vi "Teleop.vi"(10 "Match Info":T3={"Autonomous Elapsed Seconds"=0.0, "TeleOp Elapsed Seconds"=0.0, "Disabled Elapsed Seconds"=0.0, "Visited Autonomous"=FALSE, "Visited TeleOp"=FALSE, "Visited Disabled"=FALSE, "Autonomous Settings"={"Autonomous Style"=enum."Independent", "VI Refnum"=refnum}}, 11 "Call Context":T4) -> ()   [LabVIEW 2012]
doc: "This VI is called for each TeleOp packet received from the DS where the robot is not disabled. It is often used to read from the joysticks and update I/O or to update setpoints for timed control loops. It should complete and return within 20 milliseconds or it may miss DS packets."
uses:
  <vilib>/Rock Robotics/WPI/DriverStation/WPI_DriverStationDerivedRobotMode.ctl
  <vilib>/Rock Robotics/WPI/DriverStation/WPI_DriverStationMatch Info.ctl
  Control 1.ctl
  Robot Global Data.vi
  <vilib>/addons/control/pid/pid.llb/PID Output Rate Limiter (DBL).vi
  <vilib>/Rock Robotics/WPI/Joystick/WPI_JoystickGetSetRefNum.vi
  <vilib>/ptbypt/NI_PtbyPt.lvlib
  <vilib>/addons/control/pid/NI_PID_pid.lvlib
panel:
  in  "rate":dbl=500.0 format="%.2f"
  in  "ShooterTolerance":dbl=35.0
  out "RPM":dbl
  out "Pitch":dbl
  out "Enum":enum16{"Move Motor", "Engaged", "Disengaged"}(ring)
  in  "Break Disengaged":i32
  in  "Retract SH":dbl=-0.1
  in  "Time to retract motor":dbl=0.2
  in  "Break Engaged":i32=120
  in  "Test Pitch":bool
  in  "Test RPM":bool
  out "Load":bool
  in  "Reset Climb Encoder":bool
  out "Personality":string
  out "Climb Amps":dbl(graph)
  in  "sample length":i32=50
  in  "Slow Mode Divider":dbl(knob)=1.6756203903545743 scale=0.0..2.0
  in  "Elev Loop Active":bool=TRUE
  in  "Elev Bump Quanta":dbl=0.5
  out "Elev Bump":dbl
  in  "Reset Elev Bumps":bool
  out "Elevator":T1(graph)
  out "ElevatorResponse":dbl
  in  "Elevator Control (deg)":dbl(knob)=30.506718325532383 scale=15.0..40.0 scale format="%#_3g"
  in  "Reset RPM Bumps":bool
  out "RPM Bump":i64
  in  "RPM Bump Quanta":dbl=100.0
  in  "Reset Gyro":bool
  out "Climb Current":dbl
  out "Gyro Angle":dbl
  out "Elevator Encoder Volts":dbl
  out "Compressor Switch":bool
  out "Climb Encoder":dbl
  out "BB Prime":bool
  out "BB On Deck":bool
  out "Sky Hook Home":bool
  out "Drive Encoders":T1(graph)
  out "Drive Data":cluster{"Left":dbl, "Right":dbl}
  in  "Square":bool=TRUE
  in  "Which?":bool
  in  "Cheesy High & Low":T2=0.6 scale=0.0..1.0
  in  "Cheesy High":dbl(knob)=0.6 scale=0.0..1.0
  in  "Cheesy Low":dbl(knob)=0.6 scale=0.0..1.0
  in  "Quick Turn":T2=1.0 scale=0.0..1.0
  in  "Reset Encoder":bool
  out "Average Wheel Encoder":dbl
  out "Right Wheel Encoder":dbl
  out "Left Wheel Encoder":dbl
  out "Shooter RPM":cluster{dbl, "ShooterRpmResponse":dbl}(graph)
  out "Shooter RPM":dbl
  in  "Shooter RPM control":dbl(knob)=4201.533768386046 scale=0.0..5000.0
  out "Numeric 1":dbl(slide) scale=0.0..100.0
  out "Boolean 2":bool
  out "Boolean 1":bool
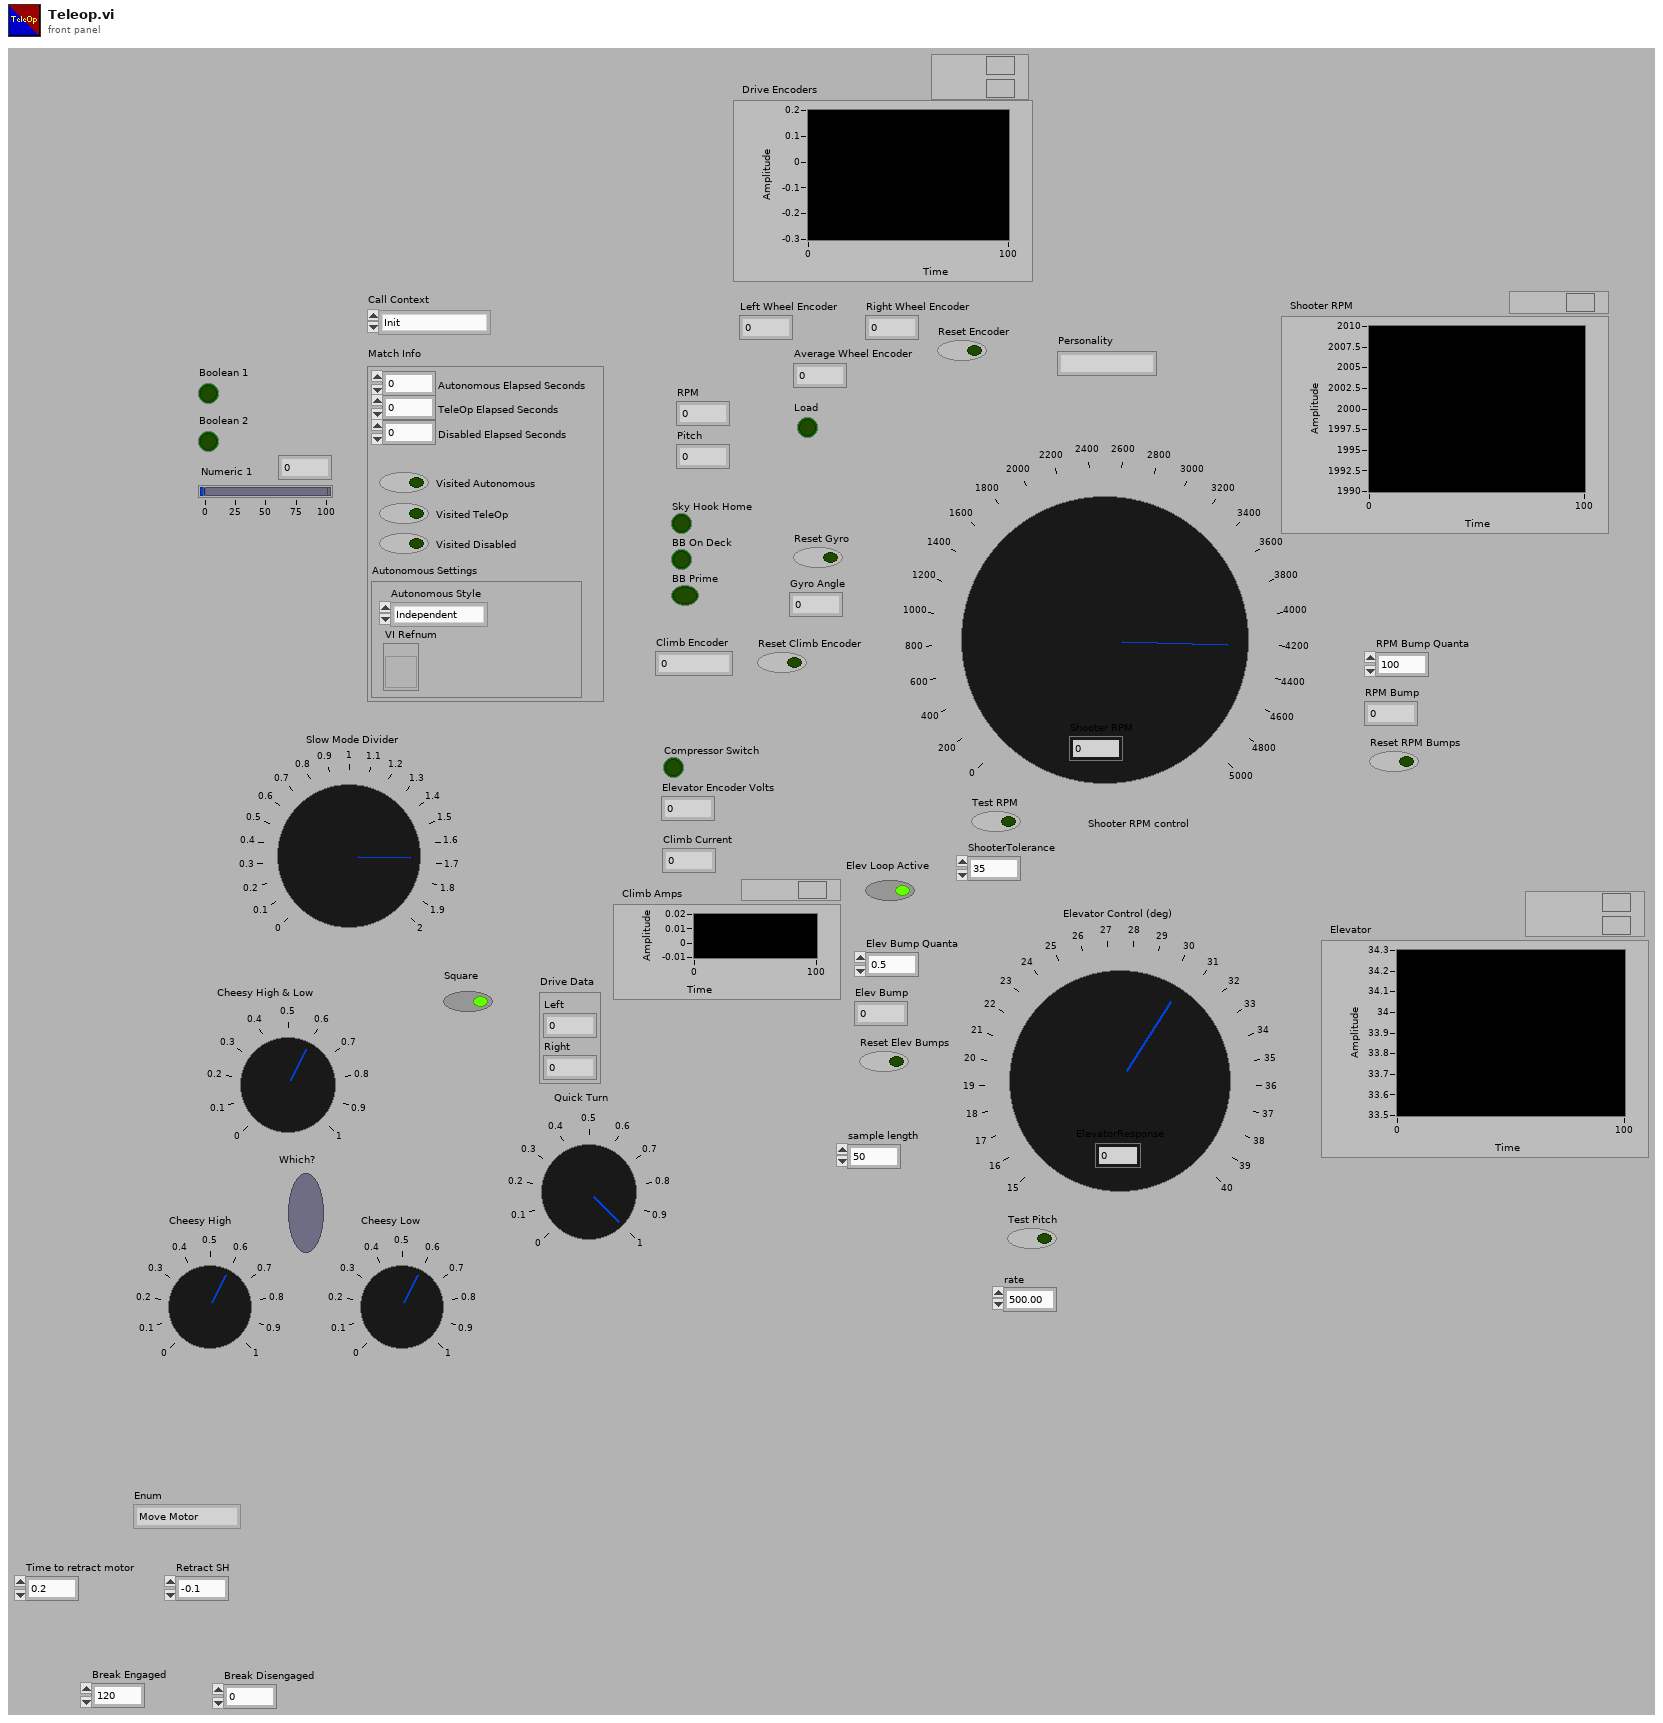
[diagram p1: front panel]
types:
  T1 = cluster{"Shooter RPM control":dbl, "ShooterRpmResponse":dbl}
  T2 = typedef "Control 1.ctl" = dbl
  T3 = typedef "WPI_DriverStationMatch Info.ctl" = cluster{"Autonomous Elapsed Seconds":dbl, "TeleOp Elapsed Seconds":dbl, "Disabled Elapsed Seconds":dbl, "Visited Autonomous":bool, "Visited TeleOp":bool, "Visited Disabled":bool, "Autonomous Settings":cluster{"Autonomous Style":enum16{"Iterative", "Independent"}, "VI Refnum":refnum<vi>}}
  T4 = typedef "WPI_DriverStationDerivedRobotMode.ctl" = enum16{"Init", "Execute", "Stop"}
  T5 = typedef "WPI_ServoDeviceRef.ctl" = cluster{"DeviceStatus":errorcluster, "Digital Module":T6, "PWM Channel":T7, "DeadBand":T8}
  T6 = typedef "FPGA_TypedefDigitalModule.ctl" = enum16{"Digital Module 1", "Digital Module 2"}
  T7 = typedef "FPGA_DIOPWMChannel.ctl" = enum8{"PWM 1", "PWM 2", "PWM 3", "PWM 4", "PWM 5", "PWM 6", "PWM 7", "PWM 8", "PWM 9", "PWM 10", "Invalid"}
  T8 = typedef "WPI_PWMDeadband.ctl" = cluster{"Name":string, "maxPositivePwm":i32, "minPositivePwm":i32, "centerPwm":i32, "maxNegativePwm":i32, "minNegativePwm":i32, "angularRange":u16}
  T9 = typedef "WPI_MotorControlDeviceRef.ctl" = cluster{"DeviceStatus":errorcluster, "Type":enum16{"PWM", "CAN"}, "PWM":cluster{"Digital Module":T6, "PWM Channel":T7, "DeadBand":T8}, "CAN":cluster{"Device Number":u8, "Control Mode":T10, "Semaphore":T11, "Max Vout":dbl}, "Invert":bool, "TransformRef":T12, "InvTransformRef":T12}
  T10 = typedef "WPI_CANJaguar_ControlMode.ctl" = enum8{"Percent VBus", "Current", "Speed", "Position", "Voltage"}
  T11 = typedef "Semaphore RefNum" = refnum<k1>
  T12 = typedef "WPI_PWMTransform_ConPane.ctl" = refnum<vi>
  T13 = typedef "WPI_JoystickDevRef.ctl" = cluster{"Device":T14}
  T14 = typedef "WPI_JoystickDeviceEnum.ctl" = enum16{"USB 1", "USB 2", "USB 3", "USB 4", "Kinect 1", "Kinect 2"}
  T15 = typedef "WPI_JoystickButtonState.ctl" = cluster{"Button 1":bool, "Button 2":bool, "Button 3":bool, "Button 4":bool, "Button 5":bool, "Button 6":bool, "Button 7":bool, "Button 8":bool, "Button 9":bool, "Button 10":bool, "Button 11":bool, "Button 12":bool}
  T16 = cluster{"axis 1 (x)":dbl, "axis 2 (y)":dbl, "axis 3 (throttle)":dbl, "axis 4":dbl, "axis 5":dbl, "axis 6":dbl}
  T17 = typedef "WPI_EncoderDevRef.ctl" = cluster{"DevStatus":errorcluster, "EncoderIndex":T18, "CounterIndex":T19, "DistancePerCount":dbl, "Decoding Type":T20}
  T18 = typedef "FPGA_EncoderIdx.ctl" = enum8{"Enc 0", "Enc 1", "Enc 2", "Enc 3", "Invalid"}
  T19 = typedef "FPGA_CounterCtrSystemIndex.ctl" = enum8{"Ctr 0", "Ctr 1", "Ctr 2", "Ctr 3", "Ctr 4", "Ctr 5", "Ctr 6", "Ctr 7", "Invalid"}
  T20 = typedef "WPI_EncoderType.ctl" = enum16{"1x", "2x", "4x"}
  T21 = typedef "WPI_DigitalInputDevRef.ctl" = cluster{"DevStatus":errorcluster, "DIO Channel":T22, "Digital Module":T6}
  T22 = typedef "FPGA_DIOChannel.ctl" = enum8{"DIO 1", "DIO 2", "DIO 3", "DIO 4", "DIO 5", "DIO 6", "DIO 7", "DIO 8", "DIO 9", "DIO 10", "DIO 11", "DIO 12", "DIO 13", "DIO 14", "Invalid"}
  T23 = typedef "WPI_AnalogChannelDevRef.ctl" = cluster{"DevStatus":errorcluster, "Analog Module":T24, "Analog Channel":T25}
  T24 = typedef "FPGA_TypedefAnalogModule.ctl" = enum16{"Analog Module 1", "Analog Module 2"}
  T25 = typedef "FPGA_AIChannel.ctl" = enum8{"AI 1", "AI 2", "AI 3", "AI 4", "AI 5", "AI 6", "AI 7", "AI 8", "Invalid"}
  T26 = typedef "WPI_GyroDevRef.ctl" = cluster{"DevStatus":errorcluster, "Analog Module":T24, "Analog Channel":T25, "Offset":dbl, "Gain (VoltsPerDegree/Second)":dbl}
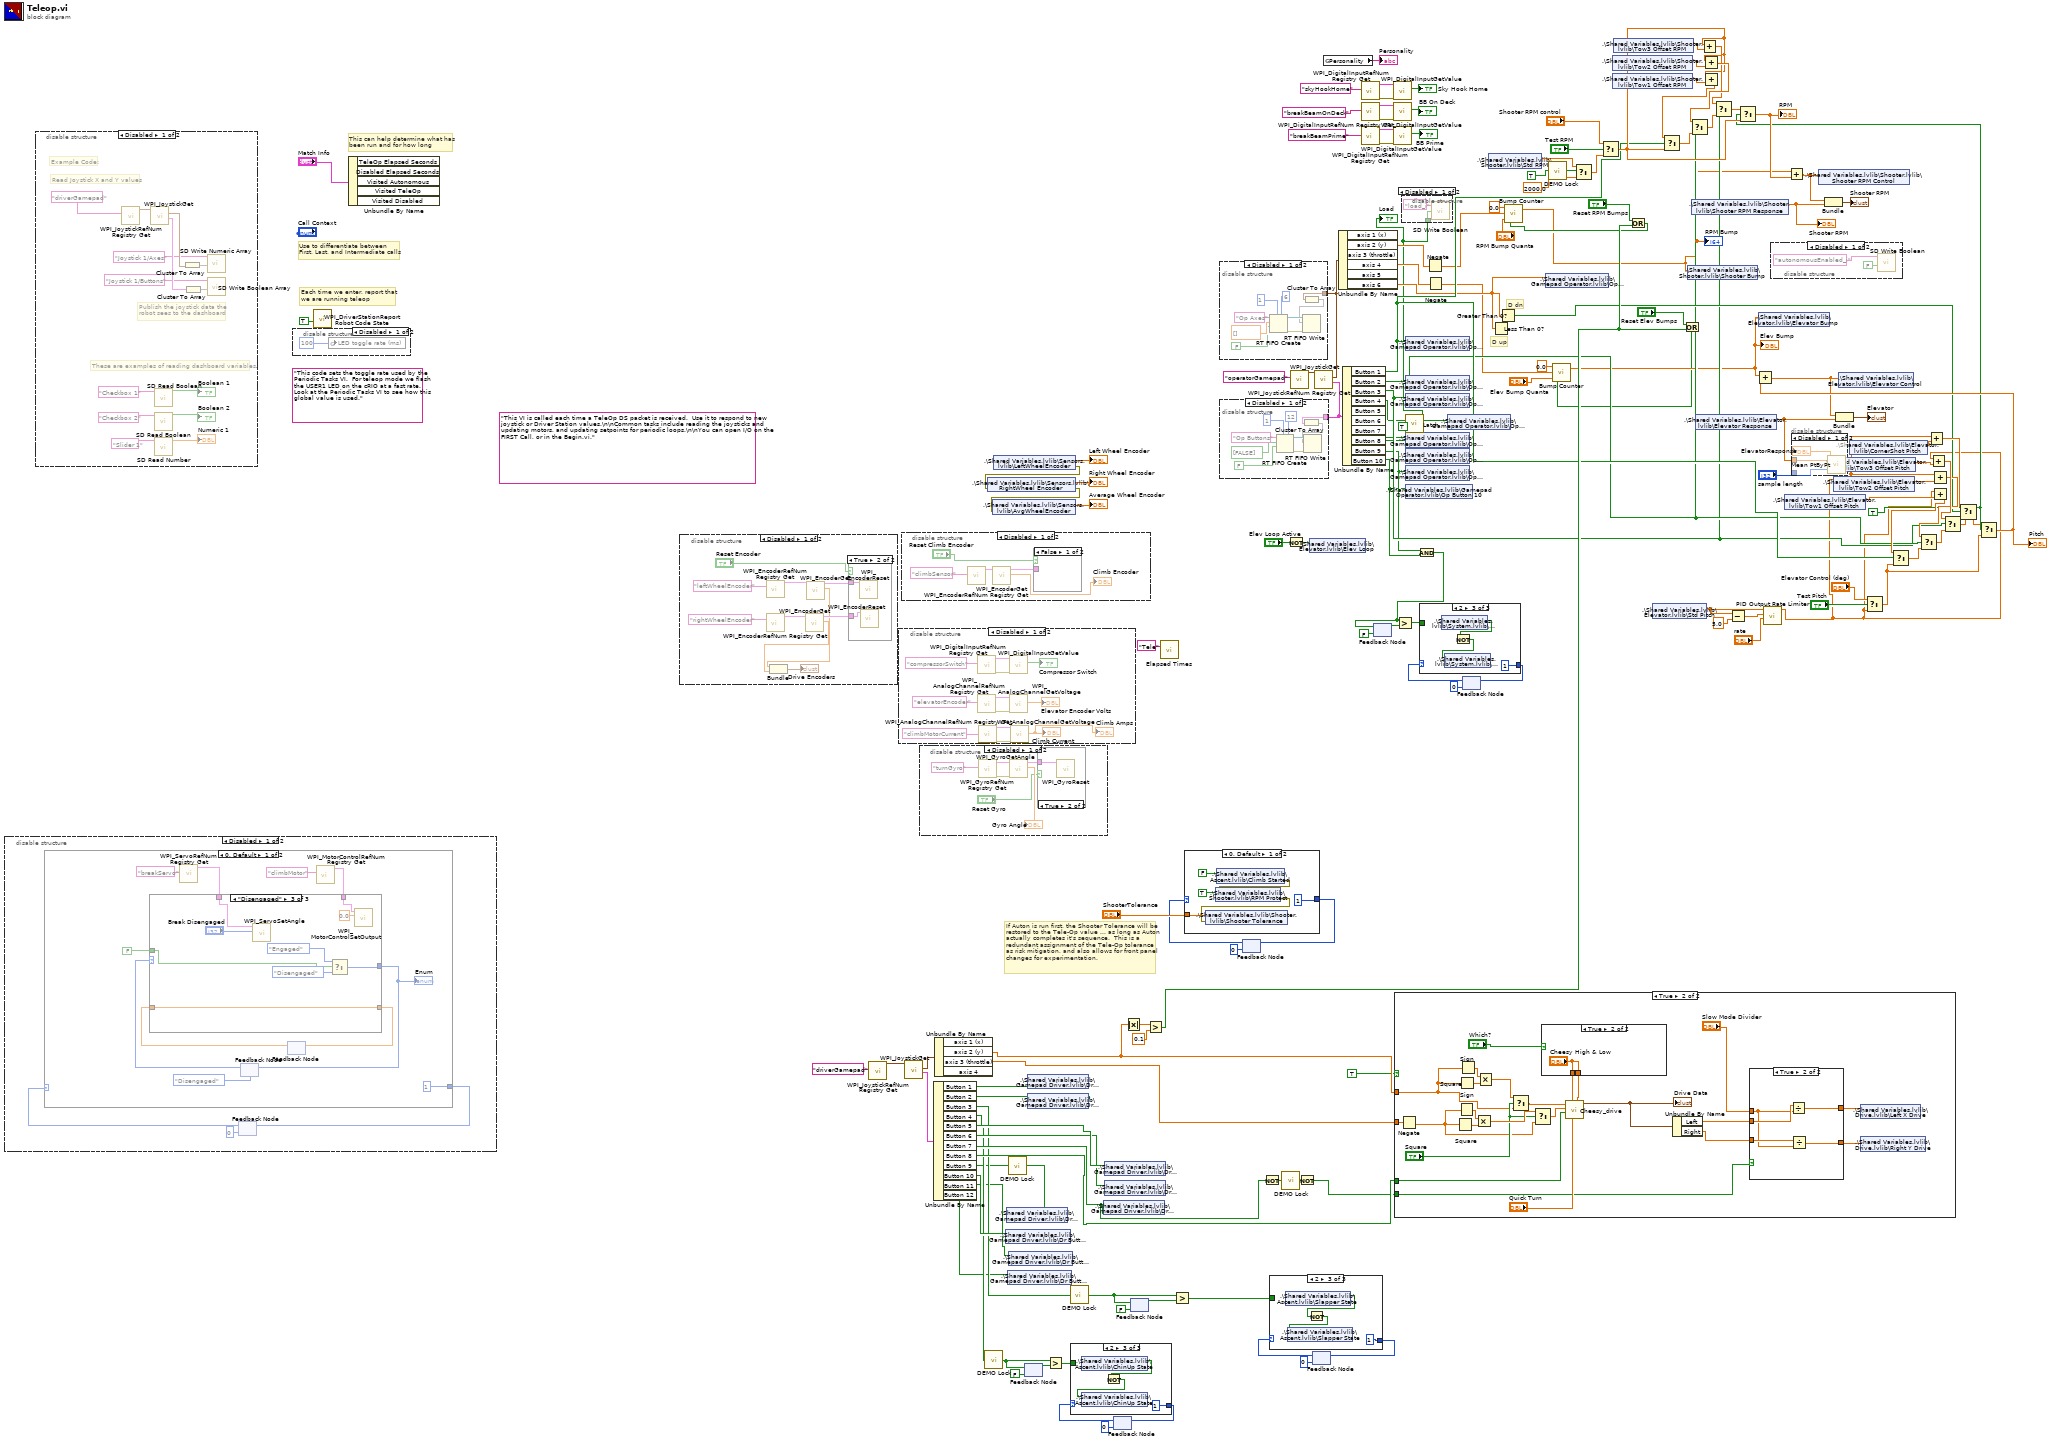
[diagram p0: block diagram]
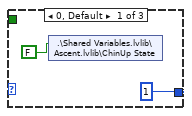
[diagram p3: hidden frame]
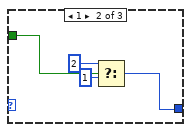
[diagram p4: hidden frame]
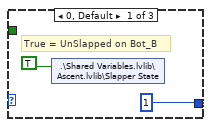
[diagram p5: hidden frame]
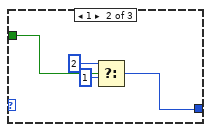
[diagram p6: hidden frame]
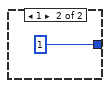
[diagram p7: hidden frame]
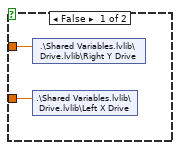
[diagram p8: hidden frame]
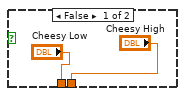
[diagram p10: hidden frame]
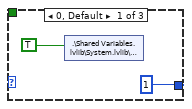
[diagram p13: hidden frame]
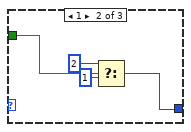
[diagram p14: hidden frame]
diagram:
  (unwired) "This code sets the toggle rate used by the Periodic Tasks VI.  For teleop mode we flash the USER1 LED on the cRIO at a fast rate.  Look at the Periodic Tasks VI to see how this global value is used."
  w115 = TRUE
  (unwired) "This VI is called each time a TeleOp DS packet is received.  Use it to respond to new joystick or Driver Station values.\n\nCommon tasks include reading the joysticks and updating motors, and updating setpoints for periodic loops.\n\nYou can open I/O on the FIRST Call, or in the Begin.vi."
  # "Each time we enter, report that\nwe are running teleop"
  # "Use to differentiate between\nFirst, Last, and Intermediate calls"
  # "This can help determine what has\nbeen run and for how long"
  # "If Auton is run first, the Shooter Tolerance will be\nrestored to the Tele-Op value ... as long as Auton\nactually completes it's sequence.  This is a\nredundant assignment of the Tele-Op tolerance\nas risk mitigation, and also allows for front panel\nchanges for experimentation."
  # "D up"
  # "D dn"
  n1 = disable-structure shown="Disabled" {
    frame Disabled {
      n2 = feedback #1(0) -> (w153:i32)
      n3 = case shown="0, Default" w153 {
        tunnel: [1 1] -> w154
        frame 0, Default {
          n4 = call <vilib>:"WPI_ServoRefNum Registry Get.vi"("refnum name"="breakServo") -> ("ServoDeviceRef"=w160:T5)  [unwired: 9 in, 1 out]
          n5 = feedback #2(enum16{"Move Motor", "Engaged", "Disengaged"}."Disengaged") -> (w165:enum16{"Move Motor", "Engaged", "Disengaged"})
          n6 = feedback #3() -> (w162:dbl)  [unwired: 1 in]
          n7 = call <vilib>:"WPI_MotorControlRefNum Registry Get.vi"("refnum name"="climbMotor") -> ("MotorControlDevRef"=w157:T9)  [unwired: 9 in, 1 out]
          n8 = case shown="\"Disengaged\"" w165 {
            tunnel: w160 -> [w174 _ w191]
            tunnel: [w168 w185 w189] -> w161
            tunnel: w162 -> [_ w185 w189]
            tunnel: [w170 w177 w195] -> w163
            tunnel: FALSE ("Break Engaged?") -> [w173 _ w190]
            tunnel: w157 -> [w167 w176 w187]
            frame "Engaged" {
              n9 = call <vilib>:"WPI_ServoSetAngle.vi"("Angle"="Break Engaged", "ServoDeviceRef"=w174) -> ()  [unwired: 8 in, 2 out]
              n10 = Select(t=enum16{"Move Motor", "Engaged", "Disengaged"}."Engaged", s=w173, f=enum16{"Move Motor", "Engaged", "Disengaged"}."Move Motor") -> (s? t:f=w170:enum16{"Move Motor", "Engaged", "Disengaged"})
              n11 = Get Date/Time In Seconds() -> (seconds since 1Jan1904=w169:timestamp)
              n12 = To Double Precision Float(number=w169) -> (double precision float=w168:dbl)
              n13 = call <vilib>:"WPI_MotorControlSetOutput.vi"("Output"=0.0, "MotorControlDevRef"=w167) -> ()  [unwired: 7 in, 3 out]
            }
            frame "Move Motor" {
              n14 = Get Date/Time In Seconds() -> (seconds since 1Jan1904=w182:timestamp)
              n15 = To Double Precision Float(number=w182) -> (double precision float=w181:dbl)
              n16 = Add(x="Time to retract motor", y=w185) -> (x+y=w184:dbl)
              n17 = Greater Or Equal?(x=w181, y=w184) -> (x >= y?=w180:bool)
              n18 = Select(t=enum16{"Move Motor", "Engaged", "Disengaged"}."Disengaged", s=w180, f=enum16{"Move Motor", "Engaged", "Disengaged"}."Move Motor") -> (s? t:f=w177:enum16{"Move Motor", "Engaged", "Disengaged"})
              n19 = call <vilib>:"WPI_MotorControlSetOutput.vi"("Output"="Retract SH", "MotorControlDevRef"=w176) -> ()  [unwired: 7 in, 3 out]
            }
            frame "Disengaged" {
              n20 = call <vilib>:"WPI_ServoSetAngle.vi"("Angle"="Break Disengaged", "ServoDeviceRef"=w191) -> ()  [unwired: 8 in, 2 out]
              n21 = Select(t=enum16{"Move Motor", "Engaged", "Disengaged"}."Engaged", s=w190, f=enum16{"Move Motor", "Engaged", "Disengaged"}."Disengaged") -> (s? t:f=w195:enum16{"Move Motor", "Engaged", "Disengaged"})
              n22 = call <vilib>:"WPI_MotorControlSetOutput.vi"("Output"=0.0, "MotorControlDevRef"=w187) -> ()  [unwired: 7 in, 3 out]
            }
          }
          "Enum" <- w163
          n23 = feedback-in #2(w163) -> ()
          n24 = feedback-in #3(w161) -> ()
        }
        frame 1 {
        }
      }
      n25 = feedback-in #1(w154) -> ()
    }
    frame Enabled {
    }
  }
  n26 = disable-structure shown="Disabled" {
    frame Disabled {
      # "Example Code:"
      # "These are examples of reading dashboard variables."
      # "Publish the joystick data the\nrobot sees to the dashboard"
      # "Read Joystick X and Y values"
      n27 = call <vilib>:"WPI_JoystickRefNum Registry Get.vi"("refnum name"="driverGamepad") -> ("JoystickDevRef"=w209:T13)  [unwired: 1 in, 9 out]
      n28 = call <vilib>:"WPI_JoystickGet.vi"("JoystickDevRef"=w209) -> ("Buttons"=w208:T15, "Axes"=w205:T16)  [unwired: 1 in, 4 out]
      n29 = call <vilib>:"SD Read Boolean.vi"("Name"="Checkbox 1" ("refnum name")) -> ("Boolean"=→"Boolean 1":bool)  [unwired: 8 in, 2 out]
      n30 = call <vilib>:"SD Read Boolean.vi"("Name"="Checkbox 2" ("refnum name")) -> ("Boolean"=→"Boolean 2":bool)  [unwired: 8 in, 2 out]
      n31 = call <vilib>:"SD Read Number.vi"("Name"="Slider 1" ("refnum name")) -> ("Numeric"=→"Numeric 1":dbl)  [unwired: 8 in, 2 out]
      n32 = Cluster To Array(cluster=w205) -> (array=w204:dbl[])
      n33 = Cluster To Array(cluster=w208) -> (array=w207:bool[])
      n34 = call <vilib>:"SD Write Numeric Array.vi"("Numeric Array"=w204, "Name"="Joystick 1/Axes") -> ()  [unwired: 8 in, 2 out]
      n35 = call <vilib>:"SD Write Boolean Array.vi"("Boolean Array"=w207, "Name"="Joystick 1/Buttons") -> ()  [unwired: 8 in, 2 out]
    }
    frame Enabled {
    }
  }
  n36 = disable-structure shown="Disabled" {
    frame Disabled {
      n37 = global write "Robot Global Data.vi" "LED toggle rate (ms)"(u32 100 ("LED ms toggle rate")) -> ()
    }
    frame Enabled {
    }
  }
  n38 = call <vilib>:"WPI_DriverStationReport Robot Code State.vi"("TeleOp"=TRUE ("Autonomous")) -> ()  [unwired: 10 in, 1 out]
  n39 = Unbundle By Name("Match Info") -> ()  [unwired: 5 out]
  n40 = disable-structure shown="Disabled" {
    frame Disabled {
      n41 = call <vilib>:"WPI_EncoderRefNum Registry Get.vi"("refnum name"="leftWheelEncoder") -> ("EncoderDevRef"=w218:T17)  [unwired: 9 in, 1 out]
      n42 = call <vilib>:"WPI_EncoderRefNum Registry Get.vi"("refnum name"="rightWheelEncoder") -> ("EncoderDevRef"=w216:T17)  [unwired: 9 in, 1 out]
      n43 = call <vilib>:"WPI_EncoderGet.vi"("EncoderDevRef"=w216) -> ("Distance"=w212:dbl, "EncoderDevRef"=w215:T17)  [unwired: 5 in, 4 out]
      n44 = call <vilib>:"WPI_EncoderGet.vi"("EncoderDevRef"=w218) -> ("Distance"=w213:dbl, "EncoderDevRef"=w217:T17)  [unwired: 5 in, 4 out]
      n45 = Bundle("Distance"=w213, "Distance"=w212) -> (→"Drive Encoders":cluster{"Distance":dbl, "Distance":dbl})  [unwired: 1 in]
      n46 = case shown="True" "Reset Encoder" {
        tunnel: w217 -> [_ w223]
        tunnel: w215 -> [_ w222]
        frame False {
        }
        frame True {
          n47 = call <vilib>:"WPI_EncoderReset.vi"("EncoderDevRef"=w223) -> ()  [unwired: 9 in, 2 out]
          n48 = call <vilib>:"WPI_EncoderReset.vi"("EncoderDevRef"=w222) -> ()  [unwired: 9 in, 2 out]
        }
      }
    }
    frame Enabled {
    }
  }
  n49 = call <vilib>:"WPI_JoystickRefNum Registry Get.vi"("refnum name"="driverGamepad") -> ("JoystickDevRef"=w55:T13)  [unwired: 9 in, 1 out]
  n50 = disable-structure shown="Disabled" {
    frame Disabled {
      n51 = call <vilib>:"WPI_DigitalInputRefNum Registry Get.vi"("refnum name"="compressorSwitch") -> ("error out"=w233:errorcluster, "DigitalInputDevRef"=w234:T21)  [unwired: 9 in]
      n52 = call <vilib>:"WPI_AnalogChannelRefNum Registry Get.vi"("refnum name"="elevatorEncoder") -> ("error out"=w231:errorcluster, "AIDeviceRef"=w230:T23)  [unwired: 9 in]
      n53 = call <vilib>:"WPI_AnalogChannelRefNum Registry Get.vi"("refnum name"="climbMotorCurrent") -> ("error out"=w226:errorcluster, "AIDeviceRef"=w227:T23)  [unwired: 9 in]
      n54 = call <vilib>:"WPI_DigitalInputGetValue.vi"("error in (no error)"=w233, "DigitalInputDevRef"=w234) -> ("Value"=→"Compressor Switch":bool)  [unwired: 7 in, 2 out]
      n55 = call <vilib>:"WPI_AnalogChannelGetVoltage.vi"("error in (no error)"=w231, "AIDeviceRef"=w230) -> ("Voltage"=→"Elevator Encoder Volts":dbl)  [unwired: 7 in, 2 out]
      n56 = call <vilib>:"WPI_AnalogChannelGetVoltage.vi"("error in (no error)"=w226, "AIDeviceRef"=w227) -> ("Voltage"=→"Climb Current" →"Climb Amps":dbl)  [unwired: 7 in, 2 out]
    }
    frame Enabled {
    }
  }
  n57 = disable-structure shown="Disabled" {
    frame Disabled {
      n58 = call <vilib>:"WPI_EncoderRefNum Registry Get.vi"("refnum name"="climbSensor") -> ("EncoderDevRef"=w240:T17)  [unwired: 9 in, 1 out]
      n59 = call <vilib>:"WPI_EncoderGet.vi"("EncoderDevRef"=w240) -> ("Distance"=→"Climb Encoder":dbl, "EncoderDevRef"=w238:T17)  [unwired: 5 in, 4 out]
      n60 = case shown="False" "Reset Climb Encoder" {
        tunnel: w238 -> [_ w241]
        frame False {
        }
        frame True {
          n61 = call <vilib>:"WPI_EncoderReset.vi"("EncoderDevRef"=w241) -> ()  [unwired: 9 in, 2 out]
        }
      }
    }
    frame Enabled {
    }
  }
  n62 = call <vilib>:"WPI_JoystickGet.vi"("JoystickDevRef"=w55) -> ("Buttons"=w52:T15, "Axes"=w53:T16)  [unwired: 4 in, 1 out]
  n63 = disable-structure shown="Disabled" {
    frame Disabled {
      n64 = call <vilib>:"WPI_GyroRefNum Registry Get.vi"("refnum name"="turnGyro") -> ("error out"=w246:errorcluster, "GyroDevRef"=w245:T26)  [unwired: 9 in]
      n65 = call <vilib>:"WPI_GyroGetAngle.vi"("error in (no error)"=w246, "GyroDevRef"=w245) -> ("Angle"=→"Gyro Angle":dbl, "GyroDevRef"=w243:T26)  [unwired: 6 in, 2 out]
      n66 = case shown="True" "Reset Gyro" {
        tunnel: w243 -> [_ w248]
        frame False {
        }
        frame True {
          n67 = call <vilib>:"WPI_GyroReset.vi"("GyroDevRef"=w248) -> ()  [unwired: 9 in, 2 out]
        }
      }
    }
    frame Enabled {
    }
  }
  n68 = Unbundle By Name(w52) -> ("Button 1"=w47:bool, "Button 2"=w46:bool, "Button 3"=w22:bool, "Button 4"=w20:bool, "Button 5"=w45:bool, "Button 6"=w44:bool, "Button 7"=w24:bool, "Button 8"=w57:bool, "Button 9"=w19:bool, "Button 10"=w43:bool, "Button 11"=w17:bool, "Button 12"=w16:bool)
  n69 = Unbundle By Name(w53) -> ("axis 2 (y)"=w56:dbl, "axis 3 (throttle)"=w58:dbl)  [unwired: 2 out]
  n70 = call "DEMO Lock.vi"("Input"=w20) -> ("Output"=w21:bool)
  n71 = shared-variable ".\\Shared Variables.lvlib\\Sensors.lvlib\\LeftWheelEncoder"() -> (→"Left Wheel Encoder":dbl, error out=w146:errorcluster)  [unwired: 1 in]
  n72 = shared-variable ".\\Shared Variables.lvlib\\Sensors.lvlib\\RightWheel Encoder"(error in=w146) -> (→"Right Wheel Encoder":dbl, error out=w145:errorcluster)
  n73 = shared-variable ".\\Shared Variables.lvlib\\Sensors.lvlib\\AvgWheelEncoder"(error in=w145) -> (→"Average Wheel Encoder":dbl)  [unwired: 1 out]
  n74 = shared-variable ".\\Shared Variables.lvlib\\Gamepad Driver.lvlib\\Dr Button 10"(w43) -> ()  [unwired: 1 in, 1 out]
  n75 = shared-variable ".\\Shared Variables.lvlib\\Gamepad Driver.lvlib\\Dr Button 12"(w16) -> ()  [unwired: 1 in, 1 out]
  n76 = shared-variable ".\\Shared Variables.lvlib\\Gamepad Driver.lvlib\\Dr Button 11"(w17) -> ()  [unwired: 1 in, 1 out]
  n77 = call "DEMO Lock.vi"("Input"=w19) -> ("Output"=w18:bool)
  n78 = shared-variable ".\\Shared Variables.lvlib\\Gamepad Driver.lvlib\\Dr Button 9"(w18) -> ()  [unwired: 1 in, 1 out]
  n79 = feedback #4(FALSE ("Button 10")) -> (w31:bool)
  n80 = feedback-in #4(w21) -> ()
  n81 = shared-variable ".\\Shared Variables.lvlib\\Gamepad Driver.lvlib\\Dr Button 1"(w47) -> ()  [unwired: 1 in, 1 out]
  n82 = shared-variable ".\\Shared Variables.lvlib\\Gamepad Driver.lvlib\\Dr Button 2"(w46) -> ()  [unwired: 1 in, 1 out]
  n83 = Greater?(x=w21, y=w31) -> (0:w33:bool)
  n84 = call "DEMO Lock.vi"("Input"=w22) -> ("Output"=w23:bool)
  n85 = shared-variable ".\\Shared Variables.lvlib\\Gamepad Driver.lvlib\\Dr Button 7"(w24) -> ()  [unwired: 1 in, 1 out]
  n86 = shared-variable ".\\Shared Variables.lvlib\\Gamepad Driver.lvlib\\Dr Button 5"(w45) -> ()  [unwired: 1 in, 1 out]
  n87 = shared-variable ".\\Shared Variables.lvlib\\Gamepad Driver.lvlib\\Dr Button 6"(w44) -> ()  [unwired: 1 in, 1 out]
  n88 = feedback #5(0) -> (w29:i32)
  n89 = case shown="2" w29 {
    tunnel: [1 w254 1 ("f")] -> w28
    tunnel: w33 -> [_ w251 _]
    frame 0, Default {
      n90 = shared-variable ".\\Shared Variables.lvlib\\Ascent.lvlib\\ChinUp State"(FALSE ("collector_override")) -> ()  [unwired: 1 in, 1 out]
    }
    frame 1 {
      n91 = Select(t=2, s=w251, f=1) -> (s? t:f=w254:i32)
    }
    frame 2 {
      n92 = shared-variable ".\\Shared Variables.lvlib\\Ascent.lvlib\\ChinUp State"() -> (w256:bool)  [unwired: 1 in, 1 out]
      n93 = Not(x=w256) -> (.not. x?=w255:bool)
      n94 = shared-variable ".\\Shared Variables.lvlib\\Ascent.lvlib\\ChinUp State"(w255) -> ()  [unwired: 1 in, 1 out]
    }
  }
  n95 = feedback-in #5(w28) -> ()
  n96 = Absolute Value(x=w56) -> (abs(x)=w51:dbl)
  n97 = feedback #6(FALSE ("Button 10")) -> (w36:bool)
  n98 = feedback-in #6(w23) -> ()
  n99 = Greater?(x=w51, y=0.1) -> (0:w151:bool)
  n100 = call "Elapsed Times.vi"("Call Name"="Tele") -> ()  [unwired: 2 in, 1 out]
  n101 = Greater?(x=w23, y=w36) -> (0:w34:bool)
  n102 = feedback #7(0) -> (w41:i32)
  n103 = case shown="0, Default" w41 {
    tunnel: [1 1] -> w42
    tunnel: "ShooterTolerance" -> [w262 _]
    frame 0, Default {
      n104 = shared-variable ".\\Shared Variables.lvlib\\Ascent.lvlib\\Climb Started"(FALSE ("Climb Started x")) -> (error out=w259:errorcluster)  [unwired: 1 in]
      n105 = shared-variable ".\\Shared Variables.lvlib\\Shooter.lvlib\\RPM Protect"(TRUE ("collector_override"), error in=w259) -> (error out=w258:errorcluster)
      n106 = shared-variable ".\\Shared Variables.lvlib\\Shooter.lvlib\\Shooter Tolerance"(w262, error in=w258) -> ()  [unwired: 1 out]
    }
    frame 1 {
    }
  }
  n107 = feedback-in #7(w42) -> ()
  n108 = Not(x=w24) -> (.not. x?=w25:bool)
  n109 = call "DEMO Lock.vi"("Input"=w25) -> ("Output"=w27:bool)
  n110 = Not(x="Elev Loop Active") -> (.not. x?=w91:bool)
  n111 = call <vilib>:"WPI_JoystickRefNum Registry Get.vi"("refnum name"="operatorGamepad") -> ("JoystickDevRef"=w142:T13)  [unwired: 9 in, 1 out]
  n112 = Not(x=w27) -> (.not. x?=w26:bool)
  n113 = shared-variable ".\\Shared Variables.lvlib\\Elevator.lvlib\\Elev Loop"(w91) -> ()  [unwired: 1 in, 1 out]
  n114 = feedback #8(0) -> (w38:i32)
  n115 = case shown="2" w38 {
    tunnel: [1 w270 1 ("f")] -> w39
    tunnel: w34 -> [_ w267 _]
    frame 0, Default {
      # "True = UnSlapped on Bot_B"
      n116 = shared-variable ".\\Shared Variables.lvlib\\Ascent.lvlib\\Slapper State"(TRUE ("collector_override")) -> ()  [unwired: 1 in, 1 out]
    }
    frame 1 {
      n117 = Select(t=2, s=w267, f=1) -> (s? t:f=w270:i32)
    }
    frame 2 {
      n118 = shared-variable ".\\Shared Variables.lvlib\\Ascent.lvlib\\Slapper State"() -> (w272:bool)  [unwired: 1 in, 1 out]
      n119 = Not(x=w272) -> (.not. x?=w271:bool)
      n120 = shared-variable ".\\Shared Variables.lvlib\\Ascent.lvlib\\Slapper State"(w271) -> ()  [unwired: 1 in, 1 out]
    }
  }
  n121 = feedback-in #8(w39) -> ()
  n122 = call <vilib>:"WPI_JoystickGet.vi"("JoystickDevRef"=w142) -> ("Buttons"=w110:T15, "Axes"=w109:T16)  [unwired: 4 in, 1 out]
  n123 = disable-structure shown="Disabled" {
    disable-tunnel: w109 -> [w282 _]
    frame Disabled {
      n124 = RT FIFO Create(0:"Op Axes" ("name (unnamed)"), 1:dbl[] [], 2:FALSE ("create if not found? (T)"), 4:u32 1 ("size (10)"), 6:u32 6 ("elements in array (1)")) -> (8:w275:refnum<k33>, 11:w276:errorcluster)  [unwired: 3 in, 1 out]
      n125 = Cluster To Array(cluster=w282) -> (array=w274:dbl[])
      n126 = RT FIFO Write(0:w275, 1:w274, 3:w276) -> ()  [unwired: 2 in, 4 out]
    }
    frame Enabled {
    }
  }
  n127 = disable-structure shown="Disabled" {
    disable-tunnel: w110 -> [w291 _]
    frame Disabled {
      n128 = RT FIFO Create(0:"Op Buttons" ("name (unnamed)"), 1:bool[] [FALSE], 2:FALSE ("create if not found? (T)"), 4:u32 1 ("size (10)"), 6:u32 12 ("elements in array (1)")) -> (8:w284:refnum<k33>, 11:w285:errorcluster)  [unwired: 3 in, 1 out]
      n129 = Cluster To Array(cluster=w291) -> (array=w283:bool[])
      n130 = RT FIFO Write(0:w284, 1:w283, 3:w285) -> ()  [unwired: 2 in, 4 out]
    }
    frame Enabled {
    }
  }
  n131 = global read "Robot Global Data.vi" "Personality"() -> (→"Personality":string)
  n132 = Unbundle By Name(w109) -> ("axis 2 (y)"=w141:dbl, "axis 4"=w140:dbl, "axis 6"=w103:dbl)  [unwired: 3 out]
  n133 = Unbundle By Name(w110) -> ("Button 1"=w108:bool, "Button 2"=w107:bool, "Button 3"=w106:bool, "Button 4"=w13:bool, "Button 6"=w105:bool, "Button 8"=w104:bool, "Button 9"=w79:bool, "Button 10"=w78:bool)  [unwired: 2 out]
  n134 = call <vilib>:"WPI_DigitalInputRefNum Registry Get.vi"("refnum name"="skyHookHome") -> ("error out"=w69:errorcluster, "DigitalInputDevRef"=w68:T21)  [unwired: 9 in]
  n135 = call <vilib>:"WPI_DigitalInputRefNum Registry Get.vi"("refnum name"="breakBeamOnDeck") -> ("error out"=w67:errorcluster, "DigitalInputDevRef"=w66:T21)  [unwired: 9 in]
  n136 = call <vilib>:"WPI_DigitalInputRefNum Registry Get.vi"("refnum name"="breakBeamPrime") -> ("error out"=w65:errorcluster, "DigitalInputDevRef"=w64:T21)  [unwired: 9 in]
  n137 = feedback #9(FALSE ("Button 10")) -> (w83:bool)
  n138 = call <vilib>:"WPI_DigitalInputGetValue.vi"("error in (no error)"=w69, "DigitalInputDevRef"=w68) -> ("Value"=→"Sky Hook Home":bool)  [unwired: 7 in, 2 out]
  n139 = call <vilib>:"WPI_DigitalInputGetValue.vi"("error in (no error)"=w67, "DigitalInputDevRef"=w66) -> ("Value"=→"BB On Deck":bool)  [unwired: 7 in, 2 out]
  n140 = call <vilib>:"WPI_DigitalInputGetValue.vi"("error in (no error)"=w65, "DigitalInputDevRef"=w64) -> ("Value"=→"BB Prime":bool)  [unwired: 7 in, 2 out]
  n141 = case shown="True" TRUE {
    tunnel: w57 -> [_ w308]
    tunnel: w56 -> [w292 w306]
    tunnel: w58 -> [w293 w304]
    tunnel: w26 -> [_ w296]
    frame False {
      n142 = shared-variable ".\\Shared Variables.lvlib\\Drive.lvlib\\Right Y Drive"(w292) -> ()  [unwired: 1 in, 1 out]
      n143 = shared-variable ".\\Shared Variables.lvlib\\Drive.lvlib\\Left X Drive"(w293) -> ()  [unwired: 1 in, 1 out]
    }
    frame True {
      n144 = Negate(x=w304) -> (-x=w305:dbl)
      n145 = Square(x=w305) -> (x^2=w314:dbl)
      n146 = Sign(1:w305) -> (0:w313:dbl)
      n147 = Square(x=w306) -> (x^2=w315:dbl)
      n148 = Sign(1:w306) -> (0:w316:dbl)
      n149 = Multiply(x=w313, y=w314) -> (x*y=w310:dbl)
      n150 = Multiply(x=w316, y=w315) -> (x*y=w309:dbl)
      n151 = Select(t=w309, s="Square", f=w306) -> (s? t:f=w311:dbl)
      n152 = Select(t=w310, s="Square", f=w305) -> (s? t:f=w312:dbl)
      n153 = case shown="True" "Which?" {
        tunnel: ["Cheesy Low" "Cheesy High & Low"] -> w302
        tunnel: ["Cheesy High" "Cheesy High & Low"] -> w301
        frame False {
        }
        frame True {
        }
      }
      n154 = call "Cheesy_drive.vi"("Speedturn_Sens_Low max"=w301, "Quickturn_Sens_Low"="Quick Turn", "Speedturn_Sens_Low"=w302, "Quick Turn"=w308, "Wheel"=w312, "Throttle"=w311) -> ("Drive Data"=w317:cluster{"Left":dbl, "Right":dbl})  [unwired: 5 in]
      "Drive Data" <- w317
      n155 = Unbundle By Name(w317) -> ("Left"=w299:dbl, "Right"=w298:dbl)
      n156 = case shown="True" w296 {
        tunnel: [w319 w324] -> w295
        tunnel: [w318 w323] -> w294
        tunnel: w299 -> [w319 w322]
        tunnel: w298 -> [w318 w321]
        tunnel: "Slow Mode Divider" -> [_ w320]
        frame False {
        }
        frame True {
          n157 = Divide(x=w322, y=w320) -> (x/y=w324:dbl)
          n158 = Divide(x=w321, y=w320) -> (x/y=w323:dbl)
        }
      }
      n159 = shared-variable ".\\Shared Variables.lvlib\\Drive.lvlib\\Left X Drive"(w295) -> ()  [unwired: 1 in, 1 out]
      n160 = shared-variable ".\\Shared Variables.lvlib\\Drive.lvlib\\Right Y Drive"(w294) -> ()  [unwired: 1 in, 1 out]
    }
  }
  n161 = call "Latch.vi"("Edge"=TRUE, "In"=w13) -> ("Out"=w12:bool)
  "Load" <- w12
  n162 = disable-structure shown="Disabled" {
    disable-tunnel: w12 -> [w328 _]
    frame Disabled {
      n163 = call <vilib>:"SD Write Boolean.vi"("Boolean"=w328, "Name"="load_i") -> ()  [unwired: 8 in, 2 out]
    }
    frame Enabled {
    }
  }
  n164 = shared-variable ".\\Shared Variables.lvlib\\Gamepad Operator.lvlib\\Op Button 1"(w108) -> ()  [unwired: 1 in, 1 out]
  n165 = shared-variable ".\\Shared Variables.lvlib\\Gamepad Operator.lvlib\\Op Button 2"(w107) -> ()  [unwired: 1 in, 1 out]
  n166 = shared-variable ".\\Shared Variables.lvlib\\Gamepad Operator.lvlib\\Op Button 3"(w106) -> ()  [unwired: 1 in, 1 out]
  n167 = shared-variable ".\\Shared Variables.lvlib\\Gamepad Operator.lvlib\\Op Button 6"(w105) -> ()  [unwired: 1 in, 1 out]
  n168 = shared-variable ".\\Shared Variables.lvlib\\Gamepad Operator.lvlib\\Op Button 8"(w104) -> ()  [unwired: 1 in, 1 out]
  n169 = shared-variable ".\\Shared Variables.lvlib\\Gamepad Operator.lvlib\\Op Button 9"(w79) -> ()  [unwired: 1 in, 1 out]
  n170 = shared-variable ".\\Shared Variables.lvlib\\Gamepad Operator.lvlib\\Op Button 10"(w78) -> ()  [unwired: 1 in, 1 out]
  n171 = And(x=w79, y=w78) -> (x .and. y?=w77:bool)
  n172 = feedback-in #9(w77) -> ()
  n173 = Greater?(x=w77, y=w83) -> (0:w85:bool)
  n174 = Negate(x=w141) -> (-x=w10:dbl)
  n175 = Negate(x=w140) -> (-x=w5:dbl)
  n176 = shared-variable ".\\Shared Variables.lvlib\\Gamepad Operator.lvlib\\Op Button 4"(w12) -> ()  [unwired: 1 in, 1 out]
  n177 = feedback #10(0) -> (w81:i32)
  n178 = case shown="2" w81 {
    tunnel: [1 w335 1 ("f")] -> w80
    tunnel: w85 -> [_ w332 _]
    frame 0, Default {
      n179 = shared-variable ".\\Shared Variables.lvlib\\System.lvlib\\DEMO"(TRUE ("collector_override")) -> ()  [unwired: 1 in, 1 out]
    }
    frame 1 {
      n180 = Select(t=2, s=w332, f=1) -> (s? t:f=w335:i32)
    }
    frame 2 {
      n181 = shared-variable ".\\Shared Variables.lvlib\\System.lvlib\\DEMO"() -> (w336:bool)  [unwired: 1 in, 1 out]
      n182 = Not(x=w336) -> (.not. x?=w337:bool)
      n183 = shared-variable ".\\Shared Variables.lvlib\\System.lvlib\\DEMO"(w337) -> ()  [unwired: 1 in, 1 out]
    }
  }
  n184 = feedback-in #10(w80) -> ()
  n185 = shared-variable ".\\Shared Variables.lvlib\\Shooter.lvlib\\Std RPM"() -> (w87:dbl)  [unwired: 1 in, 1 out]
  n186 = Less Than 0?(x=w103) -> ()  [unwired: 1 out]
  n187 = Greater Than 0?(x=w103) -> (x > 0?=w111:bool)
  n188 = shared-variable ".\\Shared Variables.lvlib\\Gamepad Operator.lvlib\\Op Dpad (y)"(w103) -> ()  [unwired: 1 in, 1 out]
  n189 = call "DEMO Lock.vi"("Input"=TRUE) -> ("Output"=w88:bool)
  n190 = Select(t=w87, s=w88, f=2000.0) -> (s? t:f=w90:dbl)
  n191 = Select(t="Shooter RPM control", s="Test RPM", f=w90) -> (s? t:f=w116:dbl)
  n192 = shared-variable ".\\Shared Variables.lvlib\\Shooter.lvlib\\Tow2 Offset RPM"() -> (w93:dbl)  [unwired: 1 in, 1 out]
  n193 = shared-variable ".\\Shared Variables.lvlib\\Shooter.lvlib\\Tow1 Offset RPM"() -> (w92:dbl)  [unwired: 1 in, 1 out]
  n194 = shared-variable ".\\Shared Variables.lvlib\\Shooter.lvlib\\Tow3 Offset RPM"() -> (w94:dbl)  [unwired: 1 in, 1 out]
  n195 = Or(x="Reset RPM Bumps", y=w151) -> (x .or. y?=w9:bool)
  n196 = call "Bump Counter.vi"("ref"=0.0, "cntrl"=w10, "quanta"="RPM Bump Quanta", "reset"=w9) -> ("out"=w7:dbl)  [unwired: 2 in]
  "RPM Bump" <- w7
  n197 = shared-variable ".\\Shared Variables.lvlib\\Elevator.lvlib\\Std Pitch"() -> (w74:dbl)  [unwired: 1 in, 1 out]
  n198 = Or(x="Reset Elev Bumps", y=w151) -> (x .or. y?=w1:bool)
  n199 = call "Bump Counter.vi"("ref"=0.0, "cntrl"=w5, "quanta"="Elev Bump Quanta", "reset"=w1) -> ("out"=w4:dbl)  [unwired: 2 in]
  "Elev Bump" <- w4
  n200 = shared-variable ".\\Shared Variables.lvlib\\Shooter.lvlib\\Shooter Bump"(w7) -> ()  [unwired: 1 in, 1 out]
  n201 = shared-variable ".\\Shared Variables.lvlib\\Shooter.lvlib\\Shooter RPM Response"() -> (w96:dbl)  [unwired: 1 in, 1 out]
  "Shooter RPM" <- w96
  n202 = shared-variable ".\\Shared Variables.lvlib\\Elevator.lvlib\\Elevator Response"() -> (w101:dbl)  [unwired: 1 in, 1 out]
  n203 = Add(x=w116, y=w94) -> (x+y=w121:dbl)
  n204 = Add(x=w116, y=w93) -> (x+y=w122:dbl)
  n205 = Add(x=w116, y=w92) -> (x+y=w123:dbl)
  n206 = Select(t=w123, s=w108, f=w116) -> (s? t:f=w119:dbl)
  n207 = Select(t=w122, s=w107, f=w119) -> (s? t:f=w118:dbl)
  n208 = Select(t=w121, s=w106, f=w118) -> (s? t:f=w120:dbl)
  n209 = Subtract(x=w74, y=5.0) -> (x-y=w73:dbl)
  n210 = Select(t=w120, s=w115, f=w116) -> (s? t:f=w117:dbl)
  "RPM" <- w117
  n211 = shared-variable ".\\Shared Variables.lvlib\\Elevator.lvlib\\Elevator Bump"(w4) -> ()  [unwired: 1 in, 1 out]
  n212 = call-poly <vilib>:"PID Output Rate Limiter.vi"("output rate (EGU/min)"="rate", "initial output"=w73, "input (controller output)"=w74) -> ("output"=w76:dbl)  [unwired: 5 in, 1 out]
  n213 = disable-structure shown="Disabled" {
    frame Disabled {
      n214 = call <vilib>:"SD Write Boolean.vi"("Boolean"=FALSE, "Name"="autonomousEnabled_i") -> ()  [unwired: 8 in, 2 out]
    }
    frame Enabled {
    }
  }
  n215 = shared-variable ".\\Shared Variables.lvlib\\Elevator.lvlib\\Tow1 Offset Pitch"() -> (w97:dbl)  [unwired: 1 in, 1 out]
  n216 = Add(x=w7, y=w117) -> (x+y=w95:dbl)
  n217 = disable-structure shown="Disabled" {
    disable-tunnel: "sample length" -> [w342 _]
    disable-tunnel: w101 -> [w341 _]
    frame Disabled {
      n218 = call <vilib>:"Mean PtByPt.vi"("x"=w341, "sample length"=w342) -> ("mean"=→"ElevatorResponse":dbl)  [unwired: 2 in, 1 out]
    }
    frame Enabled {
    }
  }
  n219 = shared-variable ".\\Shared Variables.lvlib\\Shooter.lvlib\\Shooter RPM Control"(w95) -> ()  [unwired: 1 in, 1 out]
  n220 = Bundle(w95, "Double"=w96) -> (→"Shooter RPM":cluster{dbl, "Double":dbl})  [unwired: 1 in]
  n221 = shared-variable ".\\Shared Variables.lvlib\\Elevator.lvlib\\Tow2 Offset Pitch"() -> (w98:dbl)  [unwired: 1 in, 1 out]
  n222 = shared-variable ".\\Shared Variables.lvlib\\Elevator.lvlib\\Tow3 Offset Pitch"() -> (w99:dbl)  [unwired: 1 in, 1 out]
  n223 = shared-variable ".\\Shared Variables.lvlib\\Elevator.lvlib\\CornerShot Pitch"() -> (w100:dbl)  [unwired: 1 in, 1 out]
  n224 = Select(t="Elevator Control (deg)", s="Test Pitch", f=w76) -> (s? t:f=w128:dbl)
  n225 = Add(x=w76, y=w100) -> (x+y=w112:dbl)
  n226 = Add(x=w76, y=w99) -> (x+y=w126:dbl)
  n227 = Add(x=w76, y=w98) -> (x+y=w125:dbl)
  n228 = Add(x=w76, y=w97) -> (x+y=w124:dbl)
  n229 = Select(t=w124, s=w108, f=w128) -> (s? t:f=w129:dbl)
  n230 = Select(t=w125, s=w107, f=w129) -> (s? t:f=w130:dbl)
  n231 = Select(t=w126, s=w106, f=w130) -> (s? t:f=w114:dbl)
  n232 = Select(t=w112, s=w111, f=w114) -> (s? t:f=w113:dbl)
  n233 = Select(t=w113, s=w115, f=w128) -> (s? t:f=w127:dbl)
  "Pitch" <- w127
  n234 = Add(x=w4, y=w127) -> (x+y=w102:dbl)
  n235 = Bundle(w102, "Double"=w101) -> (→"Elevator":cluster{dbl, "Double":dbl})  [unwired: 1 in]
  n236 = shared-variable ".\\Shared Variables.lvlib\\Elevator.lvlib\\Elevator Control"(w102) -> ()  [unwired: 1 in, 1 out]
